vi "main_reactor_display.vi"(3 "Env. Ready?":refnum<vi>, 5 "Storage?":refnum<vi>, 6 "Feedback?":refnum<vi>, 7 "Methane?":refnum<vi>, 8 "#Hydrolysis":refnum<vi>, 9 "Running?":refnum<vi>, 10 "Plant Picture":refnum<vi>, 11 "Reactor State":refnum<vi>) -> ()   [LabVIEW 2019]
uses:
  <vilib>/picture/picture.llb/imagedata.ctl
  lib/libSimulationControl/libSimulationControl.lvlib
panel:
  # "*******************************************************************\nBiogas Plant Control\n\nAuthor: Paul Zügel\nGCSC-Frankfurt am Main 2020\n\n*******************************************************************"
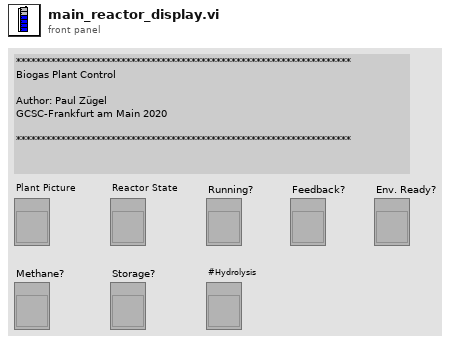
[diagram p1: front panel]
types:
  T1 = typedef "imagedata.ctl" = cluster{"image type":i32, "image depth":i32, "image":u8[], "mask":u8[], "colors":u32[], "Rectangle":cluster{"left":i16, "top":i16, "right":i16, "bottom":i16}}
  T2 = typedef "LVBoundsTypeDef.ctl" = cluster{"Width":u32, "Height":u32}
  T3 = cluster{"left":i16, "top":i16, "right":i16, "bottom":i16}
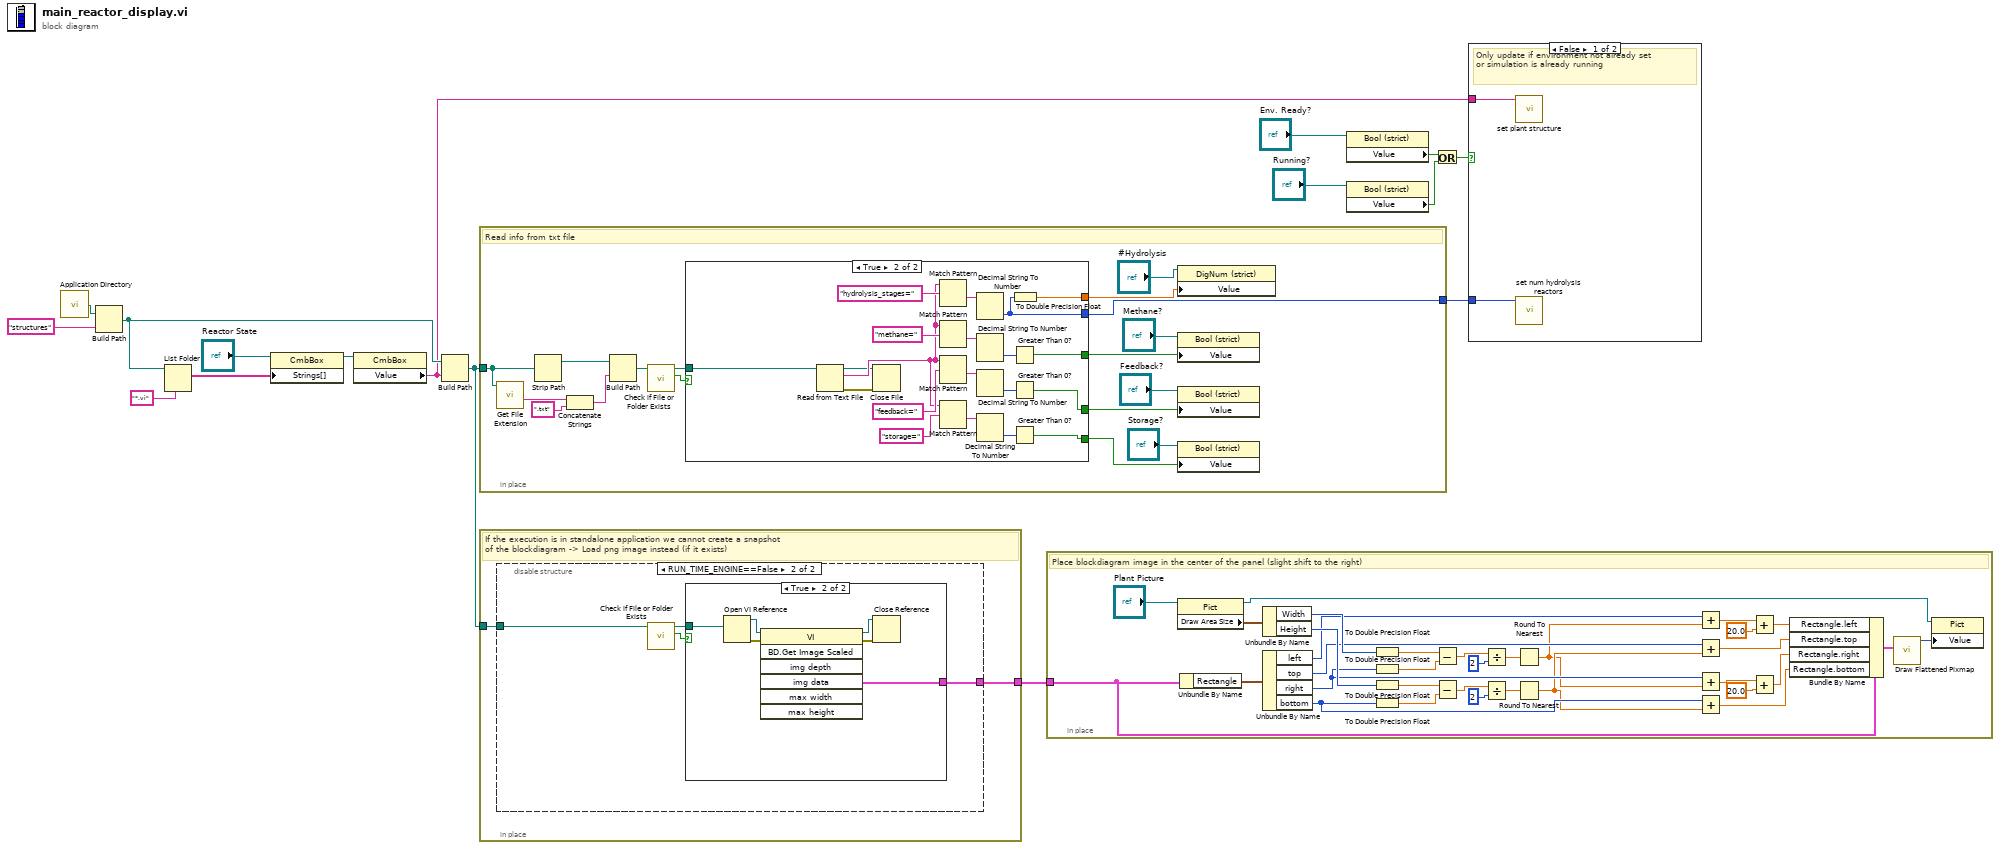
[diagram p0: block diagram]
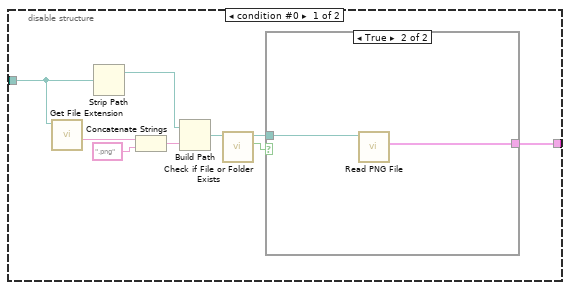
[diagram p2: hidden frame]
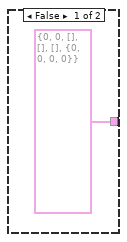
[diagram p3: hidden frame]
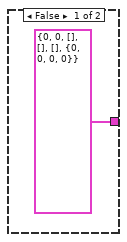
[diagram p4: hidden frame]
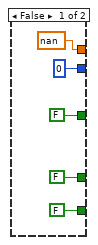
[diagram p5: hidden frame]
diagram:
  n1 = call <vilib>:"Application Directory.vi"() -> ("Application Directory"=w12:path)
  n2 = Build Path(base path=w12, name or relative path="structures") -> (appended path=w15:path)
  n3 = List Folder(path=w15, pattern="*.vi") -> (filenames=w13:string[])  [unwired: 2 in, 3 out]
  n4 = property class="CmbBox"(reference="Reactor State", "Strings[]"=w13) -> (reference out=w16:refnum<vi>)  [unwired: 1 in, 1 out]
  n5 = property class="CmbBox"(reference=w16) -> ("Value"=w8:string)  [unwired: 1 in, 2 out]
  n6 = Build Path(base path=w15, name or relative path=w8) -> (appended path=w7:path)
  n7 = in-place {
    in-place-border: w7 -> [w20]
    in-place-border: [w19] -> w6
    # "Read info from txt file"
    n8 = call <vilib>:"Get File Extension.vi"("file"=w20) -> ("filename without extension"=w21:string)  [unwired: 6 in, 4 out]
    n9 = Strip Path(path=w20) -> (stripped path=w33:path)  [unwired: 1 out]
    n10 = Concatenate Strings(w21, ".txt" ("string")) -> (w22:string)
    n11 = Build Path(base path=w33, name or relative path=w22) -> (appended path=w32:path)
    n12 = call <vilib>:"Check if File or Folder Exists.vi"("path"=w32) -> ("file or folder exists?"=w31:bool, "dup path"=w30:path)  [unwired: 8 in, 1 out]
    n13 = case shown="True" w31 {
      tunnel: w30 -> [_ w58]
      tunnel: [nan w42] -> w28
      tunnel: [FALSE ("Value") w53] -> w25
      tunnel: [FALSE ("Value") w48] -> w24
      tunnel: [0 w41] -> w19
      tunnel: [FALSE w43] -> w17
      frame False {
      }
      frame True {
        n14 = Read from Text File(file (use dialog)=w58) -> (refnum out=w40:refnum<file>, text=w44:string, error out=w39:errorcluster)  [unwired: 3 in, 1 out]
        n15 = Close File(refnum=w40, error in=w39) -> ()  [unwired: 2 out]
        n16 = Match Pattern(string=w44, regular expression="hydrolysis_stages=") -> (after substring=w56:string)  [unwired: 1 in, 3 out]
        n17 = Match Pattern(string=w44, regular expression="methane=") -> (after substring=w50:string)  [unwired: 1 in, 3 out]
        n18 = Match Pattern(string=w44, regular expression="feedback=") -> (after substring=w46:string)  [unwired: 1 in, 3 out]
        n19 = Match Pattern(string=w44, regular expression="storage=") -> (after substring=w54:string)  [unwired: 1 in, 3 out]
        n20 = Decimal String To Number(string=w56) -> (number=w41:i32)  [unwired: 2 in, 1 out]
        n21 = Decimal String To Number(string=w50) -> (number=w49:i32)  [unwired: 2 in, 1 out]
        n22 = Decimal String To Number(string=w46) -> (number=w47:i32)  [unwired: 2 in, 1 out]
        n23 = Decimal String To Number(string=w54) -> (number=w52:i32)  [unwired: 2 in, 1 out]
        n24 = Greater Than 0?(x=w49) -> (x > 0?=w48:bool)
        n25 = Greater Than 0?(x=w47) -> (x > 0?=w43:bool)
        n26 = Greater Than 0?(x=w52) -> (x > 0?=w53:bool)
        n27 = To Double Precision Float(number=w41) -> (double precision float=w42:dbl)
      }
    }
    n28 = property on="Property Node" class="DigNum (strict)"(reference="#Hydrolysis", "Value"=w28) -> ()  [unwired: 1 in, 2 out]
    n29 = property class="Bool (strict)"(reference="Methane?", "Value"=w24) -> ()  [unwired: 1 in, 2 out]
    n30 = property on="Property Node" class="Bool (strict)"(reference="Feedback?", "Value"=w17) -> ()  [unwired: 1 in, 2 out]
    n31 = property class="Bool (strict)"(reference="Storage?", "Value"=w25) -> ()  [unwired: 1 in, 2 out]
  }
  n32 = in-place {
    in-place-border: [w60] -> w10
    in-place-border: w7 -> [w59]
    # "If the execution is in standalone application we cannot create a snapshot\nof the blockdiagram -> Load png image instead (if it exists)"
    n33 = disable-structure shown="RUN_TIME_ENGINE==False" {
      disable-tunnel: w59 -> [w64 w74]
      disable-tunnel: [w61 w73] -> w60
      frame condition #0 {
        n34 = call <vilib>:"Get File Extension.vi"("file"=w64) -> ("filename without extension"=w66:string)  [unwired: 6 in, 4 out]
        n35 = Strip Path(path=w64) -> (stripped path=w68:path)  [unwired: 1 out]
        n36 = Concatenate Strings(w66, ".png" ("string")) -> (w69:string)
        n37 = Build Path(base path=w68, name or relative path=w69) -> (appended path=w67:path)
        n38 = call <vilib>:"Check if File or Folder Exists.vi"("path"=w67) -> ("file or folder exists?"=w63:bool, "dup path"=w62:path)  [unwired: 8 in, 1 out]
        n39 = case shown="True" w63 {
          tunnel: w62 -> [_ w72]
          tunnel: [T1 {"image type"=0, "image depth"=0, "image"=[], "mask"=[], "colors"=[], "Rectangle"={"left"=0, "top"=0, "right"=0, "bottom"=0}} ("image data") w71] -> w61
          frame False {
          }
          frame True {
            n40 = call <vilib>:"Read PNG File.vi"("path to PNG file"=w72) -> ("image data"=w71:T1)  [unwired: 8 in, 2 out]
          }
        }
      }
      frame condition #1 (active) {
        n41 = call <vilib>:"Check if File or Folder Exists.vi"("path"=w74) -> ("file or folder exists?"=w75:bool, "dup path"=w76:path)  [unwired: 8 in, 1 out]
        n42 = case shown="True" w75 {
          tunnel: w76 -> [_ w81]
          tunnel: [T1 {"image type"=0, "image depth"=0, "image"=[], "mask"=[], "colors"=[], "Rectangle"={"left"=0, "top"=0, "right"=0, "bottom"=0}} ("img data") w80] -> w73
          frame False {
          }
          frame True {
            n43 = Open VI Reference(vi path=w81) -> (vi reference=w83:refnum<vi>, error out=w82:errorcluster)  [unwired: 5 in]
            n44 = invoke class="VI" method="BD.Get Image Scaled"(reference=w83, error in=w82) -> (reference out=w79:refnum<vi>, error out=w78:errorcluster, "img data"=w80:T1)  [unwired: 5 in, 4 out]
            n45 = Close Reference(reference=w79, error in (no error)=w78) -> ()  [unwired: 1 out]
          }
        }
      }
    }
  }
  n46 = in-place {
    in-place-border: w10 -> [w93]
    # "Place blockdiagram image in the center of the panel (slight shift to the right)"
    n47 = property class="Pict"(reference="Plant Picture") -> (reference out=w91:refnum<vi>, "Draw Area Size"=w96:T2)  [unwired: 1 in, 1 out]
    n48 = Unbundle By Name(w93) -> ("Rectangle"=w98:T3)
    n49 = Unbundle By Name(w96) -> ("Width"=w111:u32, "Height"=w115:u32)
    n50 = Unbundle By Name(w98) -> ("left"=w99:i16, "top"=w107:i16, "right"=w109:i16, "bottom"=w113:i16)
    n51 = To Double Precision Float(number=w111) -> (double precision float=w110:dbl)
    n52 = To Double Precision Float(number=w109) -> (double precision float=w108:dbl)
    n53 = To Double Precision Float(number=w115) -> (double precision float=w114:dbl)
    n54 = To Double Precision Float(number=w113) -> (double precision float=w112:dbl)
    n55 = Subtract(x=w110, y=w108) -> (x-y=w97:dbl)
    n56 = Subtract(x=w114, y=w112) -> (x-y=w103:dbl)
    n57 = Divide(x=w97, y=u32 2) -> (x/y=w100:dbl)
    n58 = Divide(x=w103, y=u32 2) -> (x/y=w102:dbl)
    n59 = Round To Nearest(number=w100) -> (nearest integer value=w101:dbl)
    n60 = Round To Nearest(number=w102) -> (nearest integer value=w104:dbl)
    n61 = Add(x=w99, y=w101) -> (x+y=w86:dbl)
    n62 = Add(x=w107, y=w104) -> (x+y=w105:dbl)
    n63 = Add(x=w109, y=w101) -> (x+y=w88:dbl)
    n64 = Add(x=w113, y=w104) -> (x+y=w106:dbl)
    n65 = Add(x=w86, y=20.0) -> (x+y=w84:dbl)
    n66 = Add(x=w88, y=20.0) -> (x+y=w89:dbl)
    n67 = Bundle By Name(cluster=w93, "Rectangle.left"=w84, "Rectangle.top"=w105, "Rectangle.right"=w89, "Rectangle.bottom"=w106) -> (w92:T1)
    n68 = call <vilib>:"Draw Flattened Pixmap.vi"("image data"=w92) -> ("new picture"=w116:picture)  [unwired: 8 in]
    n69 = property class="Pict"(reference=w91, "Value"=w116) -> ()  [unwired: 1 in, 2 out]
  }
  n70 = property class="Bool (strict)"(reference="Env. Ready?") -> ("Value"=w4:bool)  [unwired: 1 in, 2 out]
  n71 = property class="Bool (strict)"(reference="Running?") -> ("Value"=w3:bool)  [unwired: 1 in, 2 out]
  n72 = Or(x=w4, y=w3) -> (x .or. y?=w2:bool)
  n73 = case shown="False" w2 {
    tunnel: w8 -> [w118 _]
    tunnel: w6 -> [w117 _]
    frame False {
      # "Only update if environment not already set\nor simulation is already running"
      n74 = call "set plant structure.vi"("structure"=w118) -> ()  [unwired: 10 in, 1 out]
      n75 = call "set num hydrolysis reactors.vi"("num"=w117) -> ()  [unwired: 10 in, 1 out]
    }
    frame True {
    }
  }
